vi "shutdown.vi"(8 "error in (no error)":errorcluster, 11 "wait_ms":i32) -> (0 "error out":errorcluster, 3 "processes_remaining []":i32[](array[numeric]))   [LabVIEW 2015, in "lv-waitgroup.lvlib"]
uses:
  lv-waitgroup.lvlib
  private/_controls/waitgroup.ctl
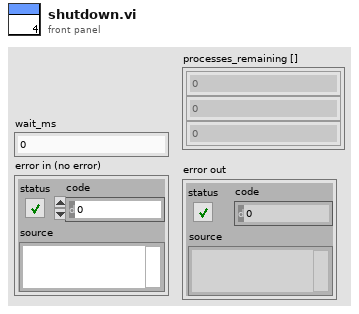
[diagram p1: front panel]
types:
  T1 = typedef "lv-waitgroup.lvlib/waitgroup.ctl" = cluster{"waitgroup":refnum<queue>, "queues":variant}
  T2 = typedef "lv-waitgroup.lvlib/references.ctl" = cluster{"waitgroups":refnum<data-value>}
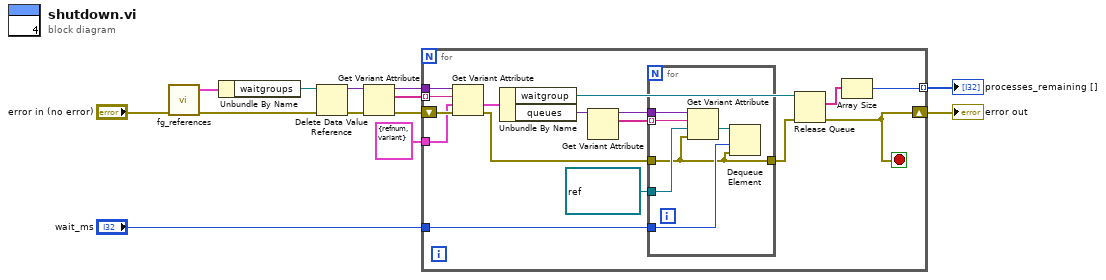
[diagram p0: block diagram]
diagram:
  n1 = call "fg_references.vi"("error in (no error)"="error in (no error)") -> ("error out"=w3:errorcluster, "references out"=w2:T2)  [unwired: 9 in]
  n2 = Unbundle By Name(w2) -> ("waitgroups"=w1:refnum<data-value>)
  n3 = Delete Data Value Reference(data value reference=w1, error in=w3) -> (data value=w13:variant, error out=w12:errorcluster)
  n4 = Get Variant Attribute(Variant=w13, error in=w12) -> (duplicate Variant=w10:variant, names=w11:string[], error out=w9:errorcluster)  [unwired: 2 in, 1 out]
  n5 = for {
    tunnel: w11 -> [w28] mode=indexing
    tunnel: w10 -> [w29]
    shift-right: [w21] -> w8
    shift-left: w9 -> [w27]
    tunnel: T1 {"waitgroup"=refnum, "queues"=variant(refnum<queue>[] [])} ("shared_data") -> [w26]
    tunnel: "wait_ms" -> [w23]
    tunnel: [w19] -> w5 mode=indexing
    stop <- w21 stop-if-true
    n6 = Get Variant Attribute(Variant=w29, name=w28, default value (empty Variant)=w26, error in=w27) -> (value=w24:T1, error out=w25:errorcluster)  [unwired: 2 out]
    n7 = Unbundle By Name(w24) -> ("waitgroup"=w14:refnum<queue>, "queues"=w18:variant)
    n8 = Get Variant Attribute(Variant=w18) -> (duplicate Variant=w16:variant, names=w17:string[])  [unwired: 3 in, 2 out]
    n9 = for {
      tunnel: w23 -> [w35]
      tunnel: w16 -> [w34]
      tunnel: w25 -> [w31]
      tunnel: [w31] -> w22
      tunnel: w17 -> [w33] mode=indexing
      tunnel: refnum<queue> refnum ("queue") -> [w32]
      n10 = Get Variant Attribute(Variant=w34, name=w33, default value (empty Variant)=w32, error in=w31) -> (value=w30:refnum<queue>)  [unwired: 3 out]
      n11 = Dequeue Element(queue=w30, timeout in ms (-1)=w35, error in (no error)=w31) -> ()  [unwired: 4 out]
    }
    n12 = Release Queue(queue=w14, error in (no error)=w22) -> (remaining elements=w20:string[], error out=w21:errorcluster)  [unwired: 1 in, 1 out]
    n13 = Array Size(array=w20) -> (size(s)=w19:i32)
  }
  "error out" <- w8
  "processes_remaining []" <- w5
